vi "RTM CreateFramesSectionChannels.vi"(8 "error in (no error)":errorcluster, 11 "Node Ptr":T1 format="%.0x") -> (0 "error out":errorcluster, 3 "Node Ptr 2":T1 format="%.0x")   [LabVIEW 2018, in "CAN Gateway System Explorer.lvlib"]
uses:
  CAN Gateway System Explorer.lvlib
  <vilib>/NI Veristand/Custom Device API/Custom Device Item Ref.ctl
  Shared/Constants.vi
  Shared/CAN Gateway Shared.lvlib
  <vilib>/NI Veristand/Custom Device API/Custom Device API.lvlib
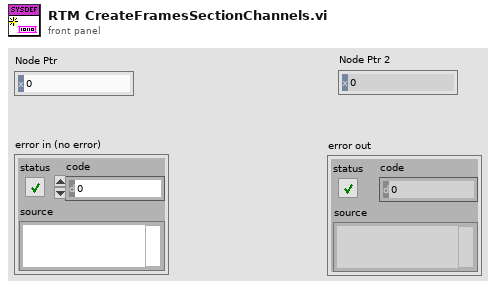
[diagram p1: front panel]
types:
  T1 = typedef "Custom Device API.lvlib/Custom Device Item Ref.ctl" = u64
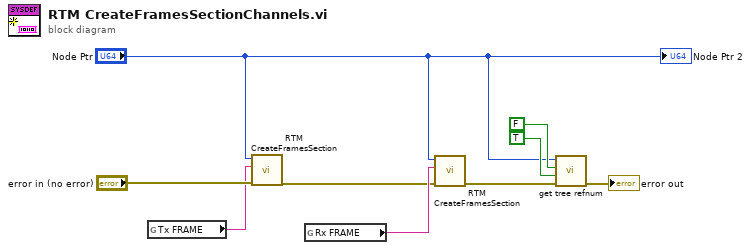
[diagram p0: block diagram]
diagram:
  n1 = global read "Constants.vi" "Tx FRAME"() -> (w8:string)
  n2 = call "RTM CreateFramesSection.vi"("error in (no error)"="error in (no error)", "Frame"=w8, "Node Ptr"="Node Ptr") -> ("error out"=w6:errorcluster)  [unwired: 7 in, 1 out]
  n3 = global read "Constants.vi" "Rx FRAME"() -> (w7:string)
  n4 = call "RTM CreateFramesSection.vi"("error in (no error)"=w6, "Frame"=w7, "Node Ptr"="Node Ptr") -> ("error out"=w2:errorcluster)  [unwired: 7 in, 1 out]
  n5 = call "get tree refnum.vi"("Error In"=w2, "Do for all Child Sections?"=TRUE, "Open?"=FALSE, "Item Ref in"="Node Ptr") -> ("Error Out"=→"error out":errorcluster)  [unwired: 6 in, 1 out]
  "Node Ptr 2" <- "Node Ptr"
